vi "NI PID Comparison.vi"() -> ()   [LabVIEW 2015]
doc: "This example demonstrates how to simulate a general PID controller."
uses:
  library/Gains.ctl
  library/Anti-Windup Method.ctl
  library/Output Range.ctl
  <vilib>/addons/control/pid/pid.llb/PID Structure.ctl
  <vilib>/addons/control/pid/pid.llb/PID Time Unit.ctl
  library/Control.vi
  library/Reset.vi
  <vilib>/addons/control/pid/pid.llb/PID Structure Conversion (DBL).vi
  <vilib>/addons/control/pid/pid.llb/PID (DBL).vi
  <vilib>/addons/control/pid/NI_PID_pid.lvlib
  library/PID.lvlib
panel:
  in  "Back-Calculation Gain Kb":dbl format="%#_13g"
  in  "Anti-Windup Method":T1
  in  "Gains":T2={"Kp"=20.0, "Ki"=0.05, "Kd"=0.0}
  out "Process Variable and Setpoint":cluster{"initial PV":dbl, "SP:":dbl}(graph)
  out "PV":dbl(slide)=60.754431603254424 scale=0.0..100.0
  out "MV":dbl(slide)=18.78965245852964 scale=-100.0..100.0
  out "Manipulated Variable":dbl(graph)
  out "NI PID Manipulated Variable":dbl(graph)
  in  "SP:":dbl(slide)=43.790849673202615 min=0.0 max=0.0 scale=0.0..100.0
  out "MV:":dbl(slide)=18.78965245852964 scale=-100.0..100.0
  out "PV:":dbl(slide)=60.754431603254424 scale=0.0..100.0
  in  "Stop":bool
  out "NI PID Process Variable and Setpoint":cluster{"initial PV":dbl, "SP:":dbl}(graph)
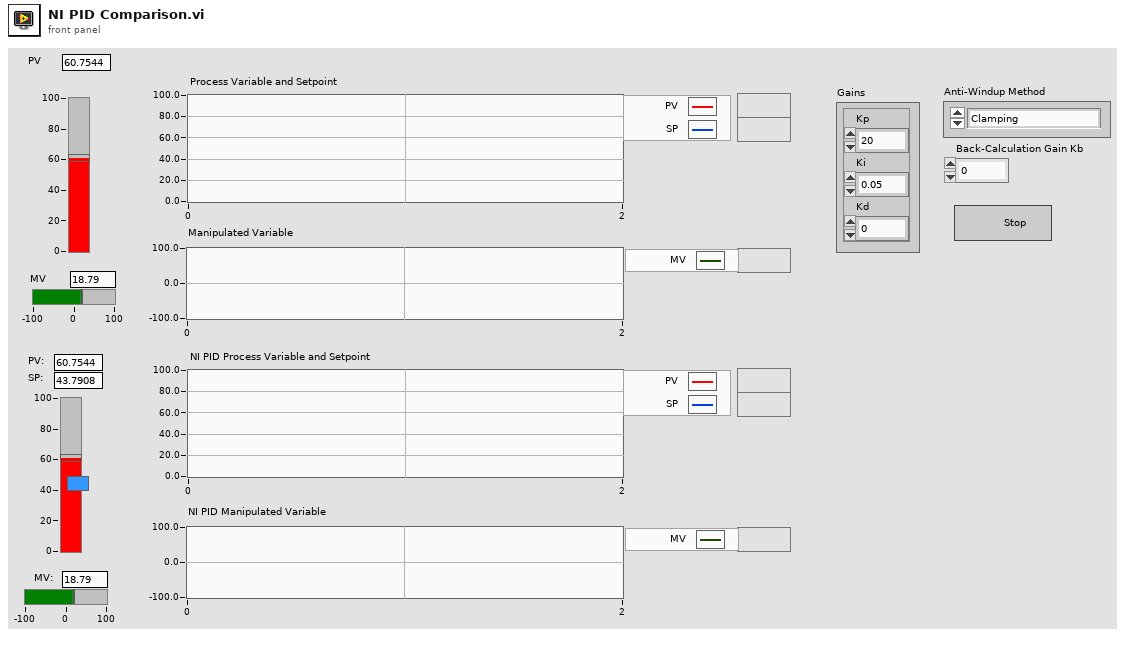
[diagram p1: front panel]
types:
  T1 = typedef "PID.lvlib/Anti-Windup Method.ctl" = enum16{"Clamping", "Back-Calculation", "None"}
  T2 = typedef "PID.lvlib/Gains.ctl" = cluster{"Kp":dbl, "Ki":dbl, "Kd":dbl}
  T3 = typedef "PID.lvlib/Output Range.ctl" = cluster{"Output Min":dbl, "Output Max":dbl}
  T4 = typedef "NI_PID_pid.lvlib/PID Time Unit.ctl" = u16
  T5 = typedef "NI_PID_pid.lvlib/PID Structure.ctl" = u16
  T6 = cluster{"static gain":dbl, "lag (min)":dbl, "dead cycles":dbl, "load %":dbl, "deadband":dbl, "noise level %":dbl, "initial PV":dbl, "initial PV 2":dbl}
  T7 = cluster{"proportional gain (Kc)":dbl, "integral time (Ti, min)":dbl, "derivative time (Td, min)":dbl}
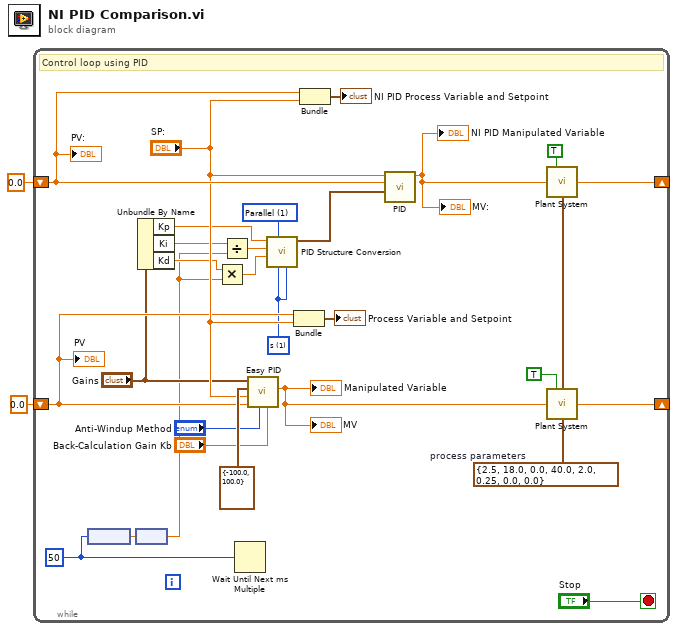
[diagram p0: block diagram]
diagram:
  n1 = while {
    shift-left: 0.0 ("Plant Output") -> [w28]
    shift-right: [w29] -> _
    shift-right: [w24] -> _
    shift-left: 0.0 ("Plant Output") -> [w18]
    stop <- "Stop" stop-if-true
    w4 = T4 1 items=["min", "s"] ("integral unit")
    w21 = T5 1 items=["Academic (Standard)", "Parallel", "Series"] ("PID structure")
    w16 = T6 {"static gain"=2.5, "lag (min)"=18.0, "dead cycles"=0.0, "load %"=40.0, "deadband"=2.0, "noise level %"=0.25, "initial PV"=0.0, "initial PV 2"=0.0}  # process parameters
    w13 = u32 50 ("unsigned 32bit integer")
    # "Control loop using PID"
    n2 = node(w13) -> (w12:dbl[unit])
    n3 = node(w12) -> (w5:dbl)
    n4 = Unbundle By Name("Gains") -> ("Kp"=w10:dbl, "Ki"=w6:dbl, "Kd"=w8:dbl)
    n5 = Multiply(x=w8, y=w5) -> (x*y=w9:dbl)
    n6 = Divide(x=w6, y=w5) -> (x/y=w7:dbl)
    n7 = Wait Until Next ms Multiple(millisecond multiple=w13) -> ()  [unwired: 1 out]
    n8 = call "Easy PID.vi"("Back-Calculation Gain Kb (1)"="Back-Calculation Gain Kb", "Anti-Windup Method (Clamping)"="Anti-Windup Method", "Process Variable"=w18, "Setpoint"="SP:", "Output Range"=T3 {"Output Min"=-100.0, "Output Max"=100.0}, "Gains"="Gains") -> ("Output"=w17:dbl)  [unwired: 5 in]
    "MV" <- w17
    "Manipulated Variable" <- w17
    n9 = call-poly <vilib>:"PID Structure Conversion.vi"("derivative unit"=w4, "integral unit"=w4, "PID structure"=w21, "derivative"=w9, "integral"=w7, "proportional"=w10) -> ("PID gains"=w20:T7)  [unwired: 5 in]
    n10 = Bundle("Plant Output"=w18, "SP:"="SP:") -> (→"Process Variable and Setpoint":cluster{"Plant Output":dbl, "SP:":dbl})  [unwired: 1 in]
    n11 = Bundle("Plant Output"=w28, "SP:"="SP:") -> (→"NI PID Process Variable and Setpoint":cluster{"Plant Output":dbl, "SP:":dbl})  [unwired: 1 in]
    n12 = call-poly <vilib>:"PID.vi"("PID gains"=w20, "process variable"=w28, "setpoint"="SP:") -> ("output"=w26:dbl)  [unwired: 7 in, 1 out]
    "MV:" <- w26
    "NI PID Manipulated Variable" <- w26
    n13 = call "Plant System.vi"("Integrator ?"=TRUE, "Plant Input"=w26, "process parameters"=w16) -> ("Plant Output"=w29:dbl)  [unwired: 12 in]
    n14 = call "Plant System.vi"("Integrator ?"=TRUE, "Plant Input"=w17, "process parameters"=w16) -> ("Plant Output"=w24:dbl)  [unwired: 12 in]
    "PV:" <- w28
    "PV" <- w18
  }
